vi "Send General Message.vi"(5 "Timestamp in message? (F)":bool, 7 "Verbose Level (1)":i32=1, 10 "error in (no error)":errorcluster, 11 "Message":string) -> (2 "error out":errorcluster)   [LabVIEW 2013, in "SET_Printf.lvlib" / "LV_Printf Msg.lvclass"]
uses:
  LV_Printf Msg.lvclass
  LV_Printf Msg.lvclass/LV_Printf Msg.ctl
  Core/LV_Printf Core.lvclass
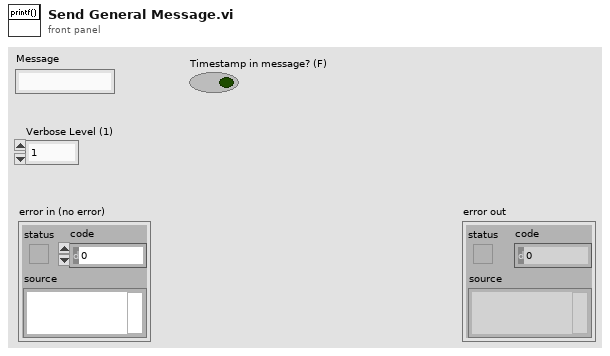
[diagram p1: front panel]
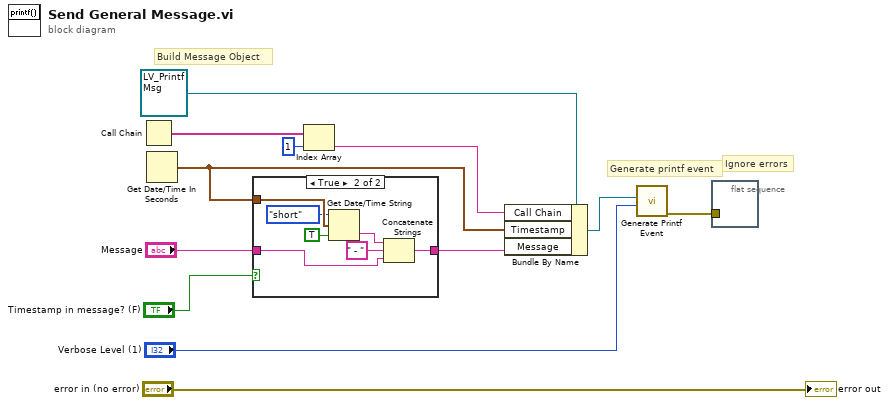
[diagram p0: block diagram]
diagram:
  # "Ignore errors"
  # "Generate printf event"
  # "Build Message Object"
  n1 = Call Chain() -> (call chain=w8:string[])
  n2 = Get Date/Time In Seconds() -> (seconds since 1Jan1904=w1:timestamp)
  n3 = case shown="True" "Timestamp in message? (F)" {
    tunnel: [w13 w20] -> w4
    tunnel: "Message" -> [w13 w14]
    tunnel: w1 -> [_ w19]
    frame False {
    }
    frame True {
      n4 = Get Date/Time String(date format (0)=enum16{"short", "long", "abbreviated"}."short", seconds (now)=w19, want seconds? (F)=TRUE) -> (time string=w16:string)  [unwired: 1 out]
      n5 = Concatenate Strings(w16, " - " ("string"), w14) -> (w20:string)
    }
  }
  n6 = Index Array(array=w8, index=1) -> (element=w6:string)
  n7 = Bundle By Name(cluster=refnum<class "LV_Printf Msg.lvclass"> refnum ("Printf_Msg_General in"), "Call Chain"=w6, "Timestamp"=w1, "Message"=w4) -> (w5:refnum<class "LV_Printf Msg.lvclass">)
  n8 = call "Generate Printf Event.vi"("Verbose Level"="Verbose Level (1)", "Printf Message"=w5) -> ("error out"=w11:errorcluster)  [unwired: 9 in]
  n9 = flat-sequence {
    tunnel: w11 -> [_]
    frame #0 {
    }
  }
  "error out" <- "error in (no error)"
